vi "启动参数设置.vi"() -> ()   [LabVIEW 2016, in "斯坦道总氮.lvlib"]
panel:
  in  "CODMn":bool
  in  "氟化物":bool
  in  "关闭":bool
  in  "保存":bool
  out "启动队列名称":cluster{"String":string, "Value":u16}[](array[cluster])
  out "启动参数":string
  in  "CODcr":bool
  in  "硫化物":bool
  in  "硅酸盐":bool
  in  "亚硝氮":bool
  in  "硝氮":bool
  in  "磷酸盐":bool
  in  "氨氮":bool
  in  "总氮":bool
  in  "总磷":bool
  # "请选择要启动的参数"
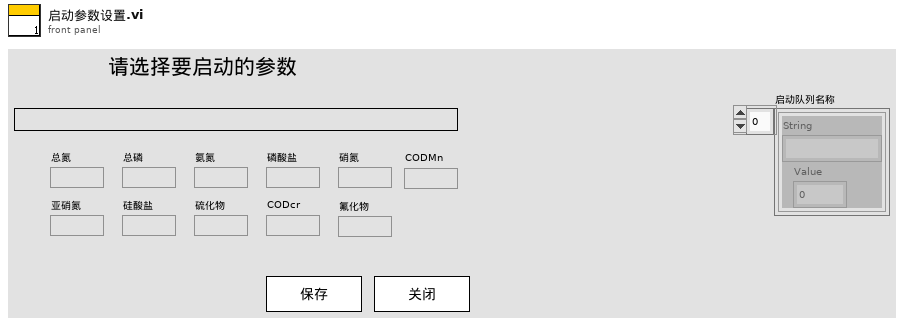
[diagram p1: front panel]
types:
  T1 = cluster{"因子编码":u32, "单位":u16, "标样参考值":sgl, "水样数据时间":timestamp, "水样实测值":sgl, "水样数据标识":string, "标样数据时间":timestamp, "标样实测值":sgl, "标样数据标识":string, "空白数据时间":timestamp, "空白实测值":sgl, "空白数据标识":string, "零点核查数据时间":timestamp, "零点核查实测值":sgl, "零点核查数据标识":string, "跨度核查数据时间":timestamp, "跨度核查实测值":sgl, "跨度核查数据标识":string, "加标回收数据时间":timestamp, "加标回收实测值":sgl, "加标回收数据标识":string, "平行样数据时间":timestamp, "平行样实测值":sgl, "平行样数据标识":string, "F0":sgl, "F1":sgl, "F2":sgl, "F3":sgl, "F4":sgl, "F5":sgl, "F6":sgl, "F7":sgl, "温度":sgl, "湿度":sgl, "X值":sgl, "fidrange":u16, "X1值":sgl}
  T2 = cluster{"测量精度":u16, "消解温度":u16, "消解时长":u16, "量程下限":sgl, "量程上限":sgl, "曲线斜率K":sgl, "曲线斜率B":sgl, "标定日期":timestamp, "标液1浓度":sgl, "标液1测量过程值":sgl, "标液2浓度":sgl, "标液2测量过程值":sgl, "标液3浓度":sgl, "标液3测量过程值":sgl, "标液4浓度":sgl, "标液4测量过程值":sgl, "标液5浓度":sgl, "标液5测量过程值":sgl, "线性相关系数":sgl, "试剂余量":u32, "测量滴定值或吸光度":sgl, "空白校准时间":timestamp, "标样校准时间":timestamp, "检出限值":sgl, "校准系数":sgl, "设备系列号":string}
  T3 = cluster{"系统时间":timestamp, "工作状态":u16, "测量模式":enum16{"待机", "连续模式", "周期模式", "定点模式", "受控模式", "手动模式"}, "告警代码":u16, "故障代码":u16, "日志代码":u16, "软件版本":u16, "F0":sgl, "F1":sgl, "F2":sgl, "F3":sgl, "T":sgl, "H":sgl, "id":u16, "flowid":u16, "量程":u16, "总磷控温温度1":sgl, "营养盐控温温度2":sgl, "ADC":sgl}
  T4 = cluster{"测量精度":u16, "消解温度":u16, "消解时长":u16, "量程下限":sgl, "量程上限":sgl, "曲线斜率K":sgl, "曲线斜率B":sgl, "标定日期":timestamp, "标液1浓度":sgl, "标液1测量过程值":sgl, "标液2浓度":sgl, "标液2测量过程值":sgl, "标液3浓度":sgl, "标液3测量过程值":sgl, "标液4浓度":sgl, "标液4测量过程值":sgl, "标液5浓度":sgl, "标液5测量过程值":sgl, "线性相关系数":sgl, "试剂余量":u32, "测量滴定值或吸光度":sgl, "空白校准时间":timestamp, "标样校准时间":timestamp, "检出限值":sgl, "校准系数":sgl, "设备系列号":string}[]
  T5 = cluster{"系统时间":timestamp, "工作状态":u16, "测量模式":enum16{"待机", "连续模式", "周期模式", "定点模式", "受控模式", "手动模式"}, "告警代码":u16, "故障代码":u16, "日志代码":u16, "软件版本":u16, "F0":sgl, "F1":sgl, "F2":sgl, "F3":sgl, "T":sgl, "H":sgl, "id":u16, "flowid":u16, "量程":u16, "总磷控温温度1":sgl, "营养盐控温温度2":sgl, "ADC":sgl}[]
  T6 = cluster{"因子编码":u32, "单位":u16, "标样参考值":sgl, "水样数据时间":timestamp, "水样实测值":sgl, "水样数据标识":string, "标样数据时间":timestamp, "标样实测值":sgl, "标样数据标识":string, "空白数据时间":timestamp, "空白实测值":sgl, "空白数据标识":string, "零点核查数据时间":timestamp, "零点核查实测值":sgl, "零点核查数据标识":string, "跨度核查数据时间":timestamp, "跨度核查实测值":sgl, "跨度核查数据标识":string, "加标回收数据时间":timestamp, "加标回收实测值":sgl, "加标回收数据标识":string, "平行样数据时间":timestamp, "平行样实测值":sgl, "平行样数据标识":string, "F0":sgl, "F1":sgl, "F2":sgl, "F3":sgl, "F4":sgl, "F5":sgl, "F6":sgl, "F7":sgl, "温度":sgl, "湿度":sgl, "X值":sgl, "fidrange":u16, "X1值":sgl}[]
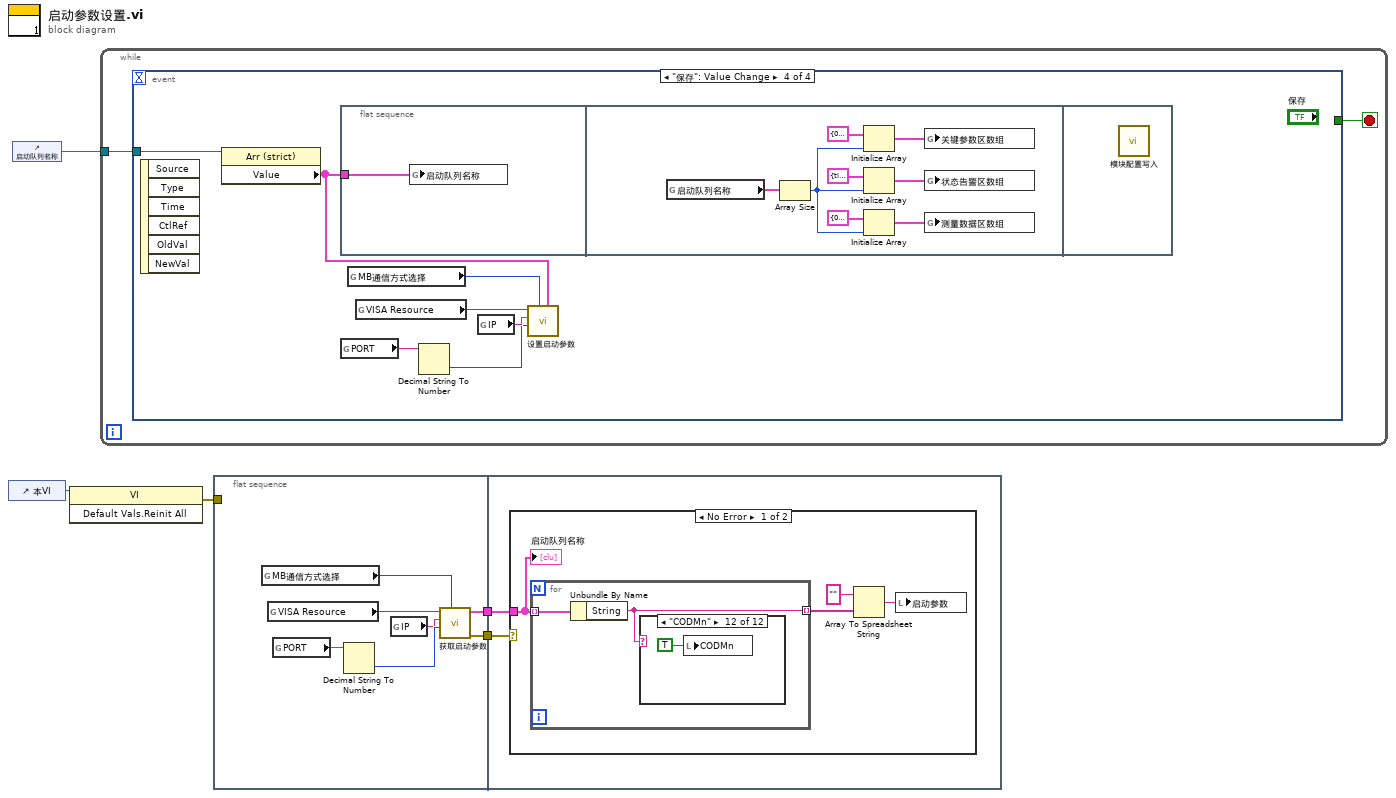
[diagram p0: block diagram]
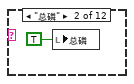
[diagram p3: hidden frame]
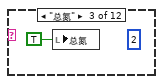
[diagram p4: hidden frame]
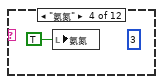
[diagram p5: hidden frame]
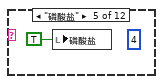
[diagram p6: hidden frame]
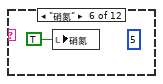
[diagram p7: hidden frame]
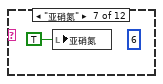
[diagram p8: hidden frame]
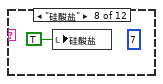
[diagram p9: hidden frame]
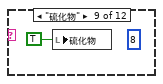
[diagram p10: hidden frame]
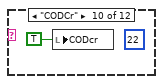
[diagram p11: hidden frame]
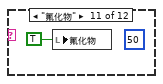
[diagram p12: hidden frame]
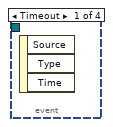
[diagram p14: hidden frame]
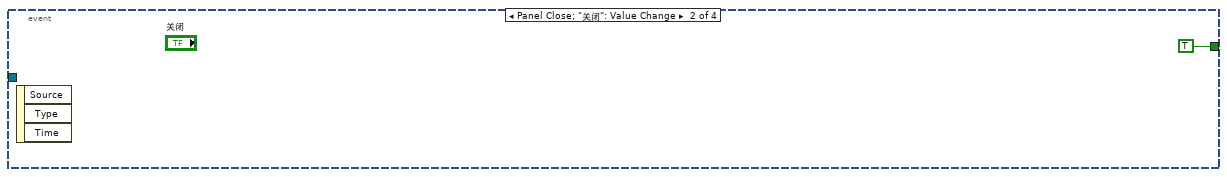
[diagram p15: hidden frame]
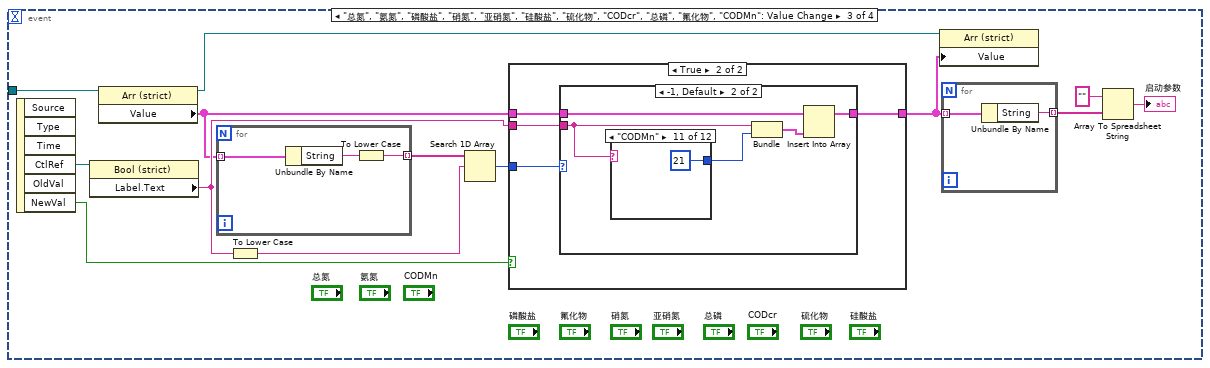
[diagram p16: hidden frame]
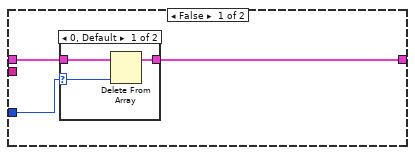
[diagram p17: hidden frame]
diagram:
  n1 = control-ref of="本VI"() -> (w4:refnum<vi>)
  n2 = control-ref of="启动队列名称"() -> (w5:refnum<vi>)
  n3 = invoke class="VI" method="Default Vals.Reinit All"(reference=w4) -> (error out=w3:errorcluster)  [unwired: 2 in, 2 out]
  n4 = while {
    tunnel: w5 -> [w6]
    stop <- w7 stop-if-true
    n5 = event shown="[3] \"保存\": Value Change" {
      selector: _ -> [_ _ _ _]
      dyn-events: _ -> [_ _ _ _]
      timeout: _ -> [_ _ _ _]
      tunnel: [_ TRUE _ _] -> w7
      tunnel: w6 -> [_ _ w13 w61]
      event Timeout {
        n6 = event-data() -> ()  [unwired: 1 in, 3 out]
      }
      event Panel Close; "关闭": Value Change {
        n7 = event-data() -> ()  [unwired: 1 in, 3 out]
      }
      event "总氮", "氨氮", "磷酸盐", "硝氮", "亚硝氮", "硅酸盐", "硫化物", "CODcr", "总磷", "氟化物", "CODMn": Value Change {
        n8 = event-data() -> ("CtlRef"=w21:refnum<vi>, "NewVal"=w20:bool)  [unwired: 1 in, 4 out]
        n9 = property class="Bool (strict)"(reference=w21) -> ("Label.Text"=w18:string)  [unwired: 1 in, 2 out]
        n10 = property class="Arr (strict)"(reference=w13) -> (reference out=w11:refnum<vi>, "Value"=w12:cluster{"String":string, "Value":u16}[])  [unwired: 1 in, 1 out]
        n11 = for {
          tunnel: w12 -> [w26] mode=indexing
          tunnel: [w24] -> w19 mode=indexing
          n12 = Unbundle By Name(w26) -> ("String"=w25:string)
          n13 = To Lower Case(string=w25) -> (all lower case string=w24:string)
        }
        n14 = To Lower Case(string=w18) -> (all lower case string=w9:string)
        n15 = Search 1D Array(1D array=w19, element=w9) -> (index of element=w17:i32)  [unwired: 1 in]
        n16 = case shown="True" w20 {
          tunnel: w18 -> [_ w36]
          tunnel: w12 -> [w28 w37]
          tunnel: w17 -> [w29 w35]
          tunnel: [w27 w34] -> w10
          frame False {
            n17 = case shown="0, Default" w29 {
              selector: w29 -> [w31 _]
              tunnel: w28 -> [w32 w33]
              tunnel: [w30 w33] -> w27
              frame 0, Default {
                n18 = Delete From Array(array=w32, index=w31) -> (array with subset deleted=w30:cluster{"String":string, "Value":u16}[])  [unwired: 1 in, 1 out]
              }
              frame -1 {
              }
            }
          }
          frame True {
            n19 = case shown="-1, Default" w35 {
              tunnel: w37 -> [w38 w43]
              tunnel: w36 -> [_ w42]
              tunnel: [w38 w39] -> w34
              frame 0 {
              }
              frame -1, Default {
                n20 = case shown="\"CODMn\"" w42 {
                  tunnel: [_ 1 2 3 4 5 6 7 8 22 21 50] -> w41
                  frame Default {
                  }
                  frame "总磷" {
                  }
                  frame "总氮" {
                  }
                  frame "氨氮" {
                  }
                  frame "磷酸盐" {
                  }
                  frame "硝氮" {
                  }
                  frame "亚硝氮" {
                  }
                  frame "硅酸盐" {
                  }
                  frame "硫化物" {
                  }
                  frame "CODCr" {
                  }
                  frame "CODMn" {
                  }
                  frame "氟化物" {
                  }
                }
                n21 = Bundle("Label.Text"=w42, w41) -> (w40:cluster{"Label.Text":string, i32})  [unwired: 1 in]
                n22 = Insert Into Array(array=w43, new element=w40) -> (w39:cluster{"String":string, "Value":u16}[])  [unwired: 1 in]
              }
            }
          }
        }
        n23 = property class="Arr (strict)"(reference=w11, "Value"=w10) -> ()  [unwired: 1 in, 2 out]
        n24 = for {
          tunnel: w10 -> [w23] mode=indexing
          tunnel: [w22] -> w16 mode=indexing
          n25 = Unbundle By Name(w23) -> ("String"=w22:string)
        }
        n26 = Array To Spreadsheet String(array=w16, 3:"" ("格式字符串")) -> (spreadsheet string=→"启动参数":string)  [unwired: 1 in]
      }
      event "保存": Value Change {
        n27 = event-data() -> ()  [unwired: 1 in, 6 out]
        n28 = property class="Arr (strict)"(reference=w61) -> ("Value"=w55:cluster{"String":string, "Value":u16}[])  [unwired: 1 in, 2 out]
        n29 = flat-sequence {
          tunnel: w55 -> [w62]
          frame #0 {
            n30 = global write "model config var.vi" "启动队列名称"(w62) -> ()
          }
          frame #1 {
            n31 = global read "model config var.vi" "启动队列名称"() -> (w64:cluster{"String":string, "Value":u16}[])
            n32 = Array Size(array=w64) -> (size(s)=w63:i32)
            n33 = Initialize Array(T2 {"测量精度"=0, "消解温度"=0, "消解时长"=0, "量程下限"=0.0, "量程上限"=0.0, "曲线斜率K"=0.0, "曲线斜率B"=0.0, "标定日期"=timestamp(0 s since 1904-01-01), "标液1浓度"=0.0, "标液1测量过程值"=0.0, "标液2浓度"=0.0, "标液2测量过程值"=0.0, "标液3浓度"=0.0, "标液3测量过程值"=0.0, "标液4浓度"=0.0, "标液4测量过程值"=0.0, "标液5浓度"=0.0, "标液5测量过程值"=0.0, "线性相关系数"=0.0, "试剂余量"=0, "测量滴定值或吸光度"=0.0, "空白校准时间"=timestamp(0 s since 1904-01-01), "标样校准时间"=timestamp(0 s since 1904-01-01), "检出限值"=0.0, "校准系数"=0.0, "设备系列号"=""} ("关键参数区"), w63) -> (w68:T4)
            n34 = Initialize Array(T3 {"系统时间"=timestamp(0 s since 1904-01-01), "工作状态"=0, "测量模式"=enum."待机", "告警代码"=0, "故障代码"=0, "日志代码"=0, "软件版本"=0, "F0"=0.0, "F1"=0.0, "F2"=0.0, "F3"=0.0, "T"=0.0, "H"=0.0, "id"=0, "flowid"=0, "量程"=0, "总磷控温温度1"=0.0, "营养盐控温温度2"=0.0, "ADC"=0.0} ("状态告警区"), w63) -> (w67:T5)
            n35 = Initialize Array(T1 {"因子编码"=0, "单位"=0, "标样参考值"=0.0, "水样数据时间"=timestamp(0 s since 1904-01-01), "水样实测值"=0.0, "水样数据标识"="", "标样数据时间"=timestamp(0 s since 1904-01-01), "标样实测值"=0.0, "标样数据标识"="", "空白数据时间"=timestamp(0 s since 1904-01-01), "空白实测值"=0.0, "空白数据标识"="", "零点核查数据时间"=timestamp(0 s since 1904-01-01), "零点核查实测值"=0.0, "零点核查数据标识"="", "跨度核查数据时间"=timestamp(0 s since 1904-01-01), "跨度核查实测值"=0.0, "跨度核查数据标识"="", "加标回收数据时间"=timestamp(0 s since 1904-01-01), "加标回收实测值"=0.0, "加标回收数据标识"="", "平行样数据时间"=timestamp(0 s since 1904-01-01), "平行样实测值"=0.0, "平行样数据标识"="", "F0"=0.0, "F1"=0.0, "F2"=0.0, "F3"=0.0, "F4"=0.0, "F5"=0.0, "F6"=0.0, "F7"=0.0, "温度"=0.0, "湿度"=0.0, "X值"=0.0, "fidrange"=0, "X1值"=0.0} ("测量数据区"), w63) -> (w70:T6)
            n36 = global write "VAR总磷总氮全局变量.vi" "关键参数区数组"(w68) -> ()
            n37 = global write "VAR总磷总氮全局变量.vi" "状态告警区数组"(w67) -> ()
            n38 = global write "VAR总磷总氮全局变量.vi" "测量数据区数组"(w70) -> ()
          }
          frame #2 {
            n39 = call "模块配置写入.vi"() -> ()  [unwired: 11 in, 1 out]
          }
        }
        n40 = global read "总磷总氮断电保存全局变量.vi" "PORT"() -> (w57:string)
        n41 = global read "总磷总氮断电保存全局变量.vi" "MB通信方式选择"() -> (w60:enum16{"串口", "TCP"})
        n42 = global read "总磷总氮断电保存全局变量.vi" "VISA Resource"() -> (w59:refnum<visa-resource-name>)
        n43 = Decimal String To Number(string=w57) -> (number=w56:i32)  [unwired: 2 in, 1 out]
        n44 = global read "总磷总氮断电保存全局变量.vi" "IP"() -> (w58:string)
        n45 = call "设置启动参数.vi"("数组"=w55, "MB通信方式选择"=w60, "Port (502)"=w56, "IP Address"=w58, "VISA Resource"=w59) -> ()  [unwired: 6 in, 1 out]
      }
    }
  }
  n46 = flat-sequence {
    tunnel: w3 -> [_]
    tunnel: [w72] -> w2
    tunnel: [w71] -> w1
    tunnel: w2 -> [w79]
    tunnel: w1 -> [w78]
    frame #0 {
      n47 = global read "总磷总氮断电保存全局变量.vi" "MB通信方式选择"() -> (w74:enum16{"串口", "TCP"})
      n48 = global read "总磷总氮断电保存全局变量.vi" "VISA Resource"() -> (w75:refnum<visa-resource-name>)
      n49 = global read "总磷总氮断电保存全局变量.vi" "PORT"() -> (w73:string)
      n50 = Decimal String To Number(string=w73) -> (number=w77:i32)  [unwired: 2 in, 1 out]
      n51 = global read "总磷总氮断电保存全局变量.vi" "IP"() -> (w76:string)
      n52 = call "获取启动参数.vi"("MB通信方式选择"=w74, "Port (502)"=w77, "IP Address"=w76, "VISA Resource"=w75) -> ("error out"=w71:errorcluster, "数组"=w72:cluster{"String":string, "Value":u16}[])  [unwired: 6 in]
    }
    frame #1 {
      n53 = case shown="No Error" w78 {
        tunnel: w79 -> [w80 _]
        frame No Error {
          n54 = for {
            tunnel: w80 -> [w85] mode=indexing
            tunnel: [w84] -> w82 mode=indexing
            n55 = Unbundle By Name(w85) -> ("String"=w84:string)
            n56 = case shown="\"CODMn\"" w84 {
              frame Default {
              }
              frame "总磷" {
                n57 = local write "总磷"(TRUE ("总磷")) -> ()
              }
              frame "总氮" {
                (unwired) 2
                n58 = local write "总氮"(TRUE ("总磷")) -> ()
              }
              frame "氨氮" {
                (unwired) 3
                n59 = local write "氨氮"(TRUE ("总磷")) -> ()
              }
              frame "磷酸盐" {
                (unwired) 4
                n60 = local write "磷酸盐"(TRUE ("总磷")) -> ()
              }
              frame "硝氮" {
                (unwired) 5
                n61 = local write "硝氮"(TRUE ("总磷")) -> ()
              }
              frame "亚硝氮" {
                (unwired) 6
                n62 = local write "亚硝氮"(TRUE ("总磷")) -> ()
              }
              frame "硅酸盐" {
                (unwired) 7
                n63 = local write "硅酸盐"(TRUE ("总磷")) -> ()
              }
              frame "硫化物" {
                (unwired) 8
                n64 = local write "硫化物"(TRUE ("总磷")) -> ()
              }
              frame "CODCr" {
                (unwired) 22
                n65 = local write "CODcr"(TRUE ("总磷")) -> ()
              }
              frame "氟化物" {
                (unwired) 50
                n66 = local write "氟化物"(TRUE ("总磷")) -> ()
              }
              frame "CODMn" {
                n67 = local write "CODMn"(TRUE ("总磷")) -> ()
              }
            }
          }
          n68 = Array To Spreadsheet String(array=w82, 3:"" ("格式字符串")) -> (spreadsheet string=w81:string)  [unwired: 1 in]
          n69 = local write "启动参数"(w81) -> ()
          "启动队列名称" <- w80
        }
        frame Error {
        }
      }
    }
  }
